vi "Label Targets3.vi"(7 "Annotate":bool=TRUE, 8 "Score Threshold":dbl, 9 "results":T1, 11 "Image in":T2) -> (3 "Image out":T2)   [LabVIEW 2019]
doc: "Draw scores near or on the particle and an ellipse around the target. Scores that are below the score threshold are drawn in red, above in green."
uses:
  <vilib>/vision/Image Controls.llb/IMAQ Image.ctl
  Target Fields.ctl
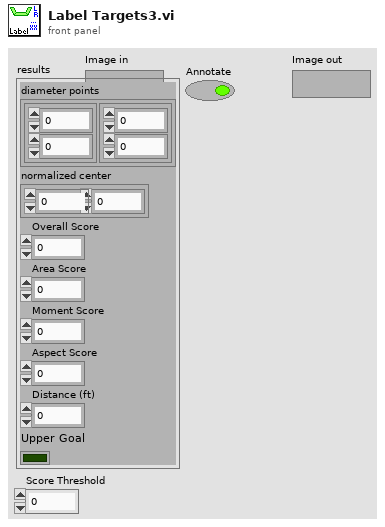
[diagram p1: front panel]
types:
  T1 = typedef "Target Fields.ctl" = cluster{"diameter points":cluster{"first point":cluster{"x":dbl, "y":dbl}, "projected point":cluster{"x":dbl, "y":dbl}}, "normalized center":cluster{"x":dbl, "y":dbl}, "Overall Score":dbl, "Area Score":dbl, "Moment Score":dbl, "Aspect Score":dbl, "Distance (ft)":dbl, "Upper Goal":bool}
  T2 = typedef "IMAQ Image.ctl" = refnum<image>
  T3 = cluster{"Desired Font (Application)":enum16{"User-specified Font", "Application Font", "System Font", "Dialog Font"}, "[User-specified Font]":cluster{"Font Name":string, "Size":i16, "Strikeout?":bool, "Italic?":bool, "Underline?":bool, "Outline?":bool, "Shadow?":bool, "Bold?":bool, "Rotation Angle":dbl}, "Horizontal Alignment":i16, "Vertical Alignment":i16}
  T4 = cluster{"first point":cluster{"x":dbl, "y":dbl}, "projected point":cluster{"x":dbl, "y":dbl}}
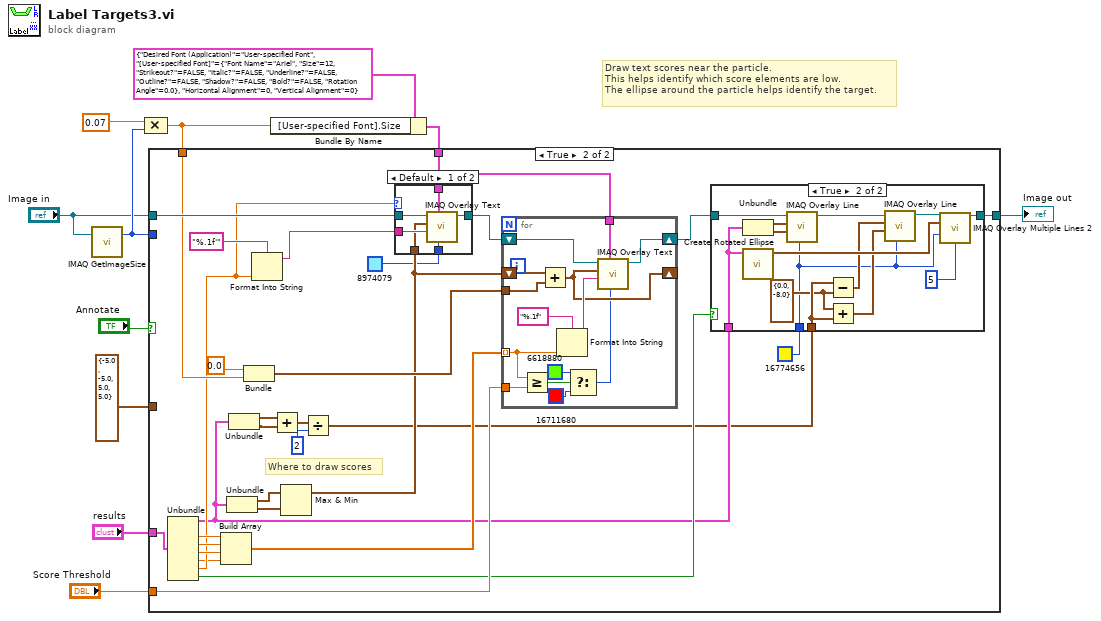
[diagram p0: block diagram]
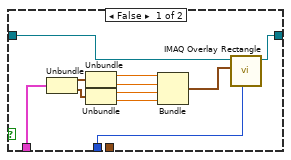
[diagram p3: hidden frame]
diagram:
  # "Draw text scores near the particle.\nThis helps identify which score elements are low.\nThe ellipse around the particle helps identify the target."
  n1 = call "IMAQ GetImageSize"("Image"="Image in") -> ("Y Resolution"=w8:i32)  [unwired: 3 in, 2 out]
  n2 = Compound Arithmetic op=MULTIPLY(0.07, w8) -> (w4:dbl)
  n3 = Bundle By Name(cluster=T3 {"Desired Font (Application)"=enum."User-specified Font", "[User-specified Font]"={"Font Name"="Ariel", "Size"=12, "Strikeout?"=FALSE, "Italic?"=FALSE, "Underline?"=FALSE, "Outline?"=FALSE, "Shadow?"=FALSE, "Bold?"=FALSE, "Rotation Angle"=0.0}, "Horizontal Alignment"=0, "Vertical Alignment"=0} ("Font, Size & Style"), "[User-specified Font].Size"=w4) -> (w5:T3)
  n4 = case shown="True" "Annotate" {
    tunnel: [w12 w36] -> w11
    tunnel: "Image in" -> [w12 w42]
    tunnel: w5 -> [_ w21]
    tunnel: w8 -> [_ _]
    tunnel: cluster{dbl, dbl, dbl, dbl} {-5.0, -5.0, 5.0, 5.0} ("output cluster") -> [_ _]
    tunnel: w4 -> [_ w38]
    tunnel: "results" -> [_ w37]
    tunnel: "Score Threshold" -> [_ w24]
    frame False {
    }
    frame True {
      # "Where to draw scores"
      n5 = Unbundle(w37) -> ("diameter points"=w18:T4, "Overall Score"=w35:dbl, "Area Score"=w34:dbl, "Moment Score"=w26:dbl, "Aspect Score"=w22:dbl, "Distance (ft)"=w23:dbl, "Upper Goal"=w20:bool)  [unwired: 1 out]
      n6 = Build Array(w35, w34, w26, w22) -> (w31:dbl[])
      n7 = Unbundle(w18) -> ("first point"=w28:cluster{"x":dbl, "y":dbl}, "projected point"=w29:cluster{"x":dbl, "y":dbl})
      n8 = Unbundle(w18) -> ("first point"=w17:cluster{"x":dbl, "y":dbl}, "projected point"=w16:cluster{"x":dbl, "y":dbl})
      n9 = Bundle(0.0, w38) -> (w30:cluster{dbl, dbl})  [unwired: 1 in]
      n10 = Format Into String(format string="%.1f'", w23) -> (resulting string=w41:string)  [unwired: 2 in, 1 out]
      n11 = Add(x=w17, y=w16) -> (x+y=w15:cluster{"x":dbl, "y":dbl})
      n12 = Max & Min(x=w28, y=w29) -> (max(x,y)=w27:cluster{"x":dbl, "y":dbl})  [unwired: 1 out]
      n13 = Divide(x=w15, y=u32 2 ("Width")) -> (x/y=w13:cluster{"x":dbl, "y":dbl})
      n14 = case shown="Default" w23 {
        tunnel: w42 -> [w87 w88]
        tunnel: w41 -> [w86 _]
        tunnel: w21 -> [w85 _]
        tunnel: [w84 w88] -> w33
        tunnel: w27 -> [w83 _]
        tunnel: u32 8974079 ("Color") -> [w82 _]
        frame Default {
          n15 = call "IMAQ Overlay Text"("Text Color (black)"=w82, "Font, Size & Style"=w85, "String"=w86, "Origin"=w83, "Image"=w87) -> ("Image Out"=w84:T2)  [unwired: 5 in, 1 out]
        }
        frame 0 {
        }
      }
      n16 = for {
        tunnel: w31 -> [w70] mode=indexing
        shift-right: [w78] -> w32
        shift-left: w33 -> [w79]
        tunnel: w21 -> [w77]
        shift-right: [w74] -> _
        shift-left: w27 -> [w75]
        tunnel: w30 -> [w76]
        tunnel: w24 -> [w69]
        n17 = Greater Or Equal?(x=w70, y=w69) -> (x >= y?=w68:bool)
        n18 = Add(x=w75, y=w76) -> (x+y=w74:cluster{dbl, dbl})
        n19 = Format Into String(format string="%.1f", w70) -> (resulting string=w80:string)  [unwired: 2 in, 1 out]
        n20 = Select(t=u32 6618880 ("Color"), s=w68, f=u32 16711680 ("Color")) -> (s? t:f=w71:u32)
        n21 = call "IMAQ Overlay Text"("Text Color (black)"=w71, "Font, Size & Style"=w77, "String"=w80, "Origin"=w74, "Image"=w79) -> ("Image Out"=w78:T2)  [unwired: 5 in, 1 out]
      }
      n22 = case shown="True" w20 {
        tunnel: [w52 w65] -> w36
        tunnel: w18 -> [w50 w62]
        tunnel: w32 -> [w53 w61]
        tunnel: u32 16774656 ("Color") -> [w51 w54]
        tunnel: w13 -> [_ w58]
        frame False {
          n23 = Unbundle(w50) -> ("first point"=w49:cluster{"x":dbl, "y":dbl}, "projected point"=w48:cluster{"x":dbl, "y":dbl})
          n24 = Unbundle(w49) -> ("x"=w47:dbl, "y"=w46:dbl)
          n25 = Unbundle(w48) -> ("x"=w45:dbl, "y"=w44:dbl)
          n26 = Bundle("x"=w47, "y"=w46, "x"=w45, "y"=w44) -> (w43:cluster{"x":dbl, "y":dbl, "x":dbl, "y":dbl})  [unwired: 1 in]
          n27 = call "IMAQ Overlay Rectangle"("Color"=w51, "Rectangle"=w43, "Image"=w53) -> ("Image Out"=w52:T2)  [unwired: 7 in, 1 out]
        }
        frame True {
          w55 = cluster{"x":dbl, "y":dbl} {"x"=0.0, "y"=-8.0} ("x/y")
          n28 = Unbundle(w62) -> ("first point"=w67:cluster{"x":dbl, "y":dbl}, "projected point"=w66:cluster{"x":dbl, "y":dbl})
          n29 = call "Create Rotated Ellipse.vi"("diameter points"=w62) -> ("XY Graph"=w64:cluster{"X":dbl, "Y":dbl}[])  [unwired: 10 in]
          n30 = call "IMAQ Overlay Line"("Color"=w54, "End Point"=w66, "Start Point"=w67, "Image"=w61) -> ("Image Out"=w60:T2)  [unwired: 6 in, 1 out]
          n31 = Subtract(x=w58, y=w55) -> (x-y=w57:cluster{"x":dbl, "y":dbl})
          n32 = Add(x=w55, y=w58) -> (x+y=w56:cluster{"x":dbl, "y":dbl})
          n33 = call "IMAQ Overlay Line"("Color"=w54, "End Point"=w56, "Start Point"=w57, "Image"=w60) -> ("Image Out"=w59:T2)  [unwired: 6 in, 1 out]
          n34 = call "IMAQ Overlay Multiple Lines 2"("Image"=w59, "Line End Points"=w64, "Color"=w54, "Width"=u32 5) -> ("Image Out"=w65:T2)  [unwired: 10 in, 1 out]
        }
      }
    }
  }
  "Image out" <- w11
